vi "Open.vi"(8 "error in (no error)":errorcluster, 11 "MelsecTCP in":refnum<class "MelsecFxLinks.lvclass">) -> (0 "error out":errorcluster, 2 "IsSuccess":bool, 3 "MelsecTCP out":refnum<class "MelsecFxLinks.lvclass">)   [LabVIEW 2020, in "MelsecFxLinks.lvclass"]
uses:
  MelsecFxLinks.lvclass
  C:/Users/Fred Guo/Desktop/API_Salcomp_CMES/Libraries/HslCommunication/HslCommunication.dll
  HslCommunication.dll
  MelsecFxLinks.lvclass/MelsecFxLinks.ctl
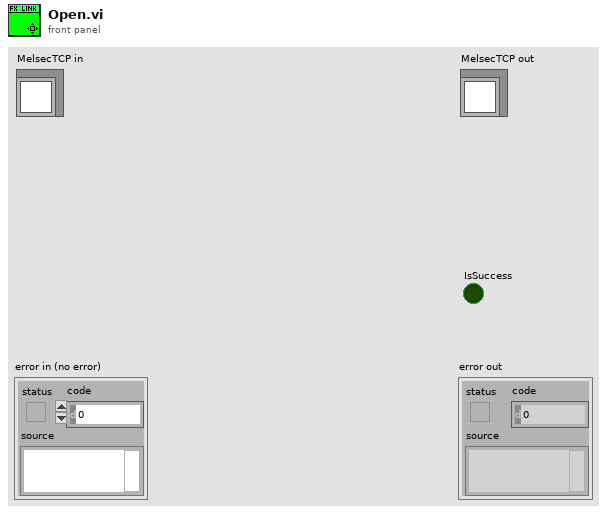
[diagram p1: front panel]
types:
  T1 = cluster{"portName":string, "baudRate":i32, "dataBits":i32, "stopBits":i32, "parity":i32}
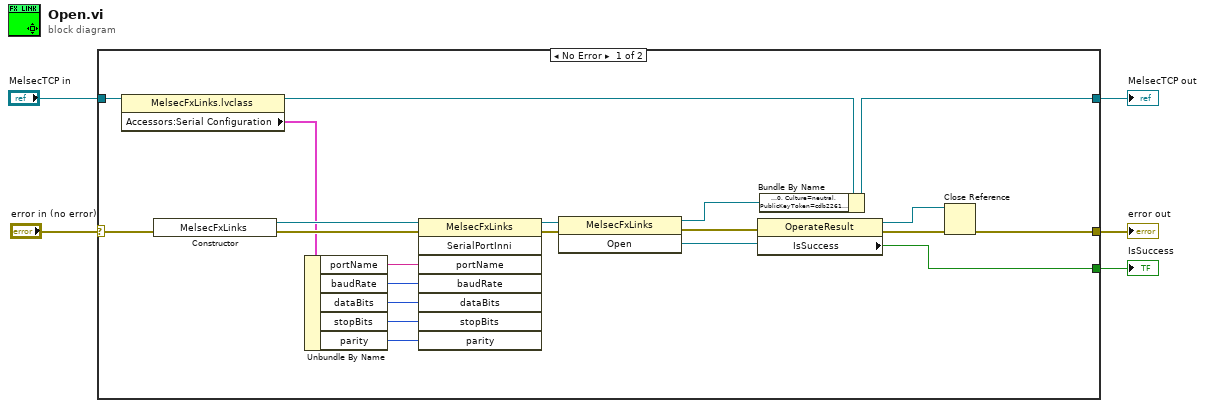
[diagram p0: block diagram]
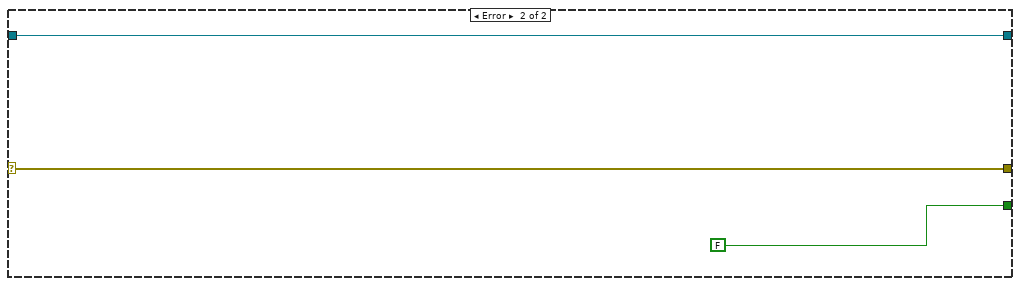
[diagram p2: hidden frame]
diagram:
  n1 = case shown="No Error" "error in (no error)" {
    selector: "error in (no error)" -> [w18 w29]
    tunnel: "MelsecTCP in" -> [w26 w28]
    tunnel: [w23 w29] -> w4
    tunnel: [w17 w28] -> w2
    tunnel: [w21 FALSE ("IsSuccess")] -> w1
    frame No Error {
      n2 = property class="MelsecFxLinks.lvclass"(reference=w26) -> (reference out=w22:refnum<class "MelsecFxLinks.lvclass">, "Accessors:Serial Configuration"=w12:T1)  [unwired: 1 in, 1 out]
      n3 = constructor class="MelsecFxLinks"(error in=w18) -> (reference out=w20:refnum<k24>, error out=w19:errorcluster)  [unwired: 2 in, 1 out]
      n4 = Unbundle By Name(w12) -> ("portName"=w7:string, "baudRate"=w8:i32, "dataBits"=w9:i32, "stopBits"=w10:i32, "parity"=w11:i32)
      n5 = invoke class="MelsecFxLinks" method="SerialPortInni"(reference=w20, error in=w19, "portName"=w7, "baudRate"=w8, "dataBits"=w9, "stopBits"=w10, "parity"=w11) -> (reference out=w16:refnum<k24>, error out=w15:errorcluster)  [unwired: 1 in, 6 out]
      n6 = invoke class="MelsecFxLinks" method="Open"(reference=w16, error in=w15) -> (reference out=w13:refnum<k24>, error out=w6:errorcluster, "Open"=w14:refnum<k24>)  [unwired: 1 in]
      n7 = property class="OperateResult"(reference=w14, error in=w6) -> (reference out=w25:refnum<k24>, error out=w24:errorcluster, "IsSuccess"=w21:bool)
      n8 = Bundle By Name(cluster=w22, "new reference"=w13) -> (w17:refnum<class "MelsecFxLinks.lvclass">)
      n9 = Close Reference(reference=w25, error in (no error)=w24) -> (error out=w23:errorcluster)
    }
    frame Error {
    }
  }
  "error out" <- w4
  "MelsecTCP out" <- w2
  "IsSuccess" <- w1
